vi "DeviceClose.vi"(4 "error in (no error)":errorcluster, 7 "CmdLib In":refnum<k24>) -> (0 "error out":errorcluster, 3 "CmdLib Out":refnum<k24>)   [LabVIEW 2013]
uses:
  C:/Code/Apps/Utilities/AG-UC2-UC8/AG-UC2-UC8/Install/Samples/LabVIEW/LabVIEW 2013/CmdLibAgilis.dll
  CmdLibAgilis.dll
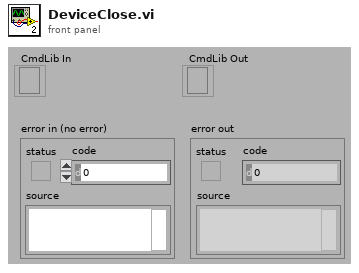
[diagram p1: front panel]
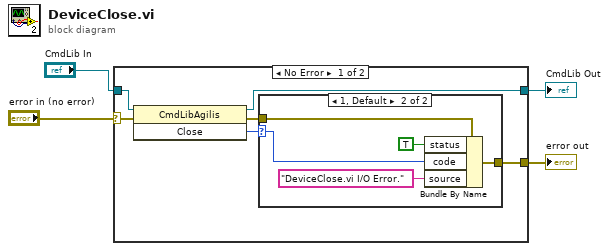
[diagram p0: block diagram]
diagram:
  n1 = case shown="No Error" "error in (no error)" {
    selector: "error in (no error)" -> [w5 w18]
    tunnel: [w7 w18] -> w3
    tunnel: "CmdLib In" -> [w10 w17]
    tunnel: [w9 w17] -> w1
    frame No Error {
      n2 = invoke class="CmdLibAgilis" method="Close"(reference=w10, error in=w5) -> (reference out=w9:refnum<k24>, error out=w6:errorcluster, "Close"=w8:i32)  [unwired: 1 in]
      n3 = case shown="1, Default" w8 {
        selector: w8 -> [_ w12]
        tunnel: w6 -> [w11 w14]
        tunnel: [w11 w13] -> w7
        frame 0 {
        }
        frame 1, Default {
          n4 = Bundle By Name(cluster=w14, "status"=TRUE, "code"=w12, "source"="DeviceClose.vi I/O Error.") -> (w13:errorcluster)
        }
      }
    }
    frame Error {
    }
  }
  "error out" <- w3
  "CmdLib Out" <- w1
